vi "Read_ini_file.vi"() -> ()   [LabVIEW 2018]
uses:
  <vilib>/Utility/config.llb/Read Key (I32).vi
  <vilib>/Utility/config.llb/Read Key (U32).vi
  <vilib>/Utility/config.llb/NI_LVConfig.lvlib
panel:
  out "appended path":path
  out "file or folder exists?":bool
  out "Pulley Position":u32
  out "Active Layer":i32
  out "error out (config.ini file)":errorcluster
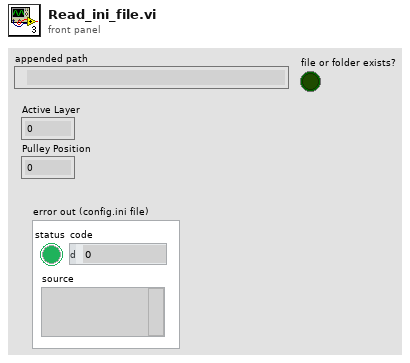
[diagram p1: front panel]
types:
  T1 = typedef "NI_LVConfig.lvlib/Config Data RefNum.ctl" = refnum<k1>
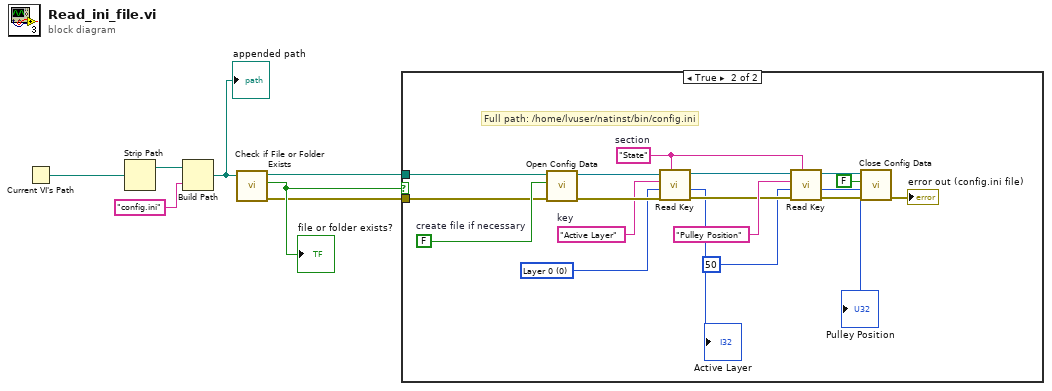
[diagram p0: block diagram]
diagram:
  n1 = Current VI's Path() -> (path=w6:path)
  n2 = Strip Path(path=w6) -> (stripped path=w7:path)  [unwired: 1 out]
  n3 = Build Path(base path=w7, name or relative path="config.ini") -> (appended path=w4:path)
  "appended path" <- w4
  n4 = call <vilib>:"Check if File or Folder Exists.vi"("path"=w4) -> ("error out"=w1:errorcluster, "file or folder exists?"=w3:bool, "dup path"=w2:path)  [unwired: 8 in]
  "file or folder exists?" <- w3
  n5 = case shown="True" w3 {
    tunnel: w2 -> [_ w9]
    tunnel: w1 -> [_ w8]
    frame False {
    }
    frame True {
      w14 = 0 items=["Layer 0", "Layer 1", "Layer 2", "Layer 3"] ("Active Layer")
      w22 = "Active Layer"  # key
      w20 = "State"  # section
      w25 = FALSE  # create file if necessary
      # "Full path: /home/lvuser/natinst/bin/config.ini"
      n6 = call <vilib>:"Open Config Data.vi"("error in (no error)"=w8, "create file if necessary (T)"=w25, "configuration file path"=w9) -> ("error out"=w23:errorcluster, "refnum"=w24:T1)  [unwired: 6 in, 1 out]
      n7 = call-poly <vilib>:"Read Key.vi"("section"=w20, "error in (no error)"=w23, "default value"=w14, "key"=w22, "refnum"=w24) -> ("error out"=w18:errorcluster, "value"=→"Active Layer":i32, "refnum out"=w21:T1)  [unwired: 3 in, 1 out]
      n8 = call-poly <vilib>:"Read Key.vi"("section"=w20, "error in (no error)"=w18, "default value"=u32 50 ("Pulley Position"), "key"="Pulley Position", "refnum"=w21) -> ("error out"=w17:errorcluster, "value"=→"Pulley Position":u32, "refnum out"=w16:T1)  [unwired: 3 in, 1 out]
      n9 = call <vilib>:"Close Config Data.vi"("error in (no error)"=w17, "write file if changed (T)"=FALSE, "refnum"=w16) -> ("error out"=→"error out (config.ini file)":errorcluster)  [unwired: 7 in, 1 out]
    }
  }
